vi "py.vi"() -> ()   [LabVIEW 2023]
panel:
  in  "x 2":dbl(slide) scale=0.0..10.0
  in  "Stop":bool
  out "Numeric":i32
  out "return value":T1
  in  "x":dbl(slide) scale=0.0..10.0
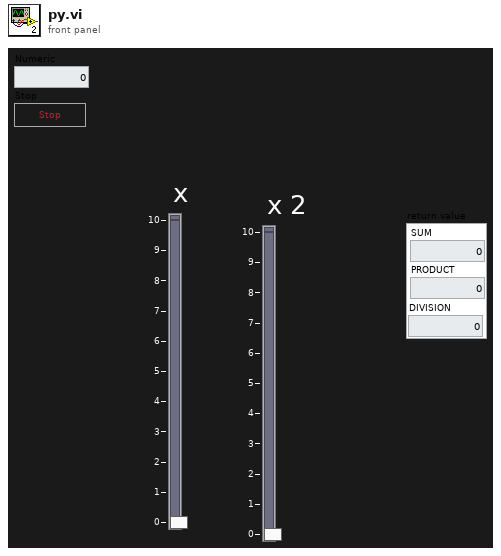
[diagram p1: front panel]
types:
  T1 = cluster{"SUM":dbl, "PRODUCT":dbl, "DIVISION":dbl}
  T2 = cluster{"Numeric":dbl, "Numeric 2":dbl, "Numeric 3":dbl}
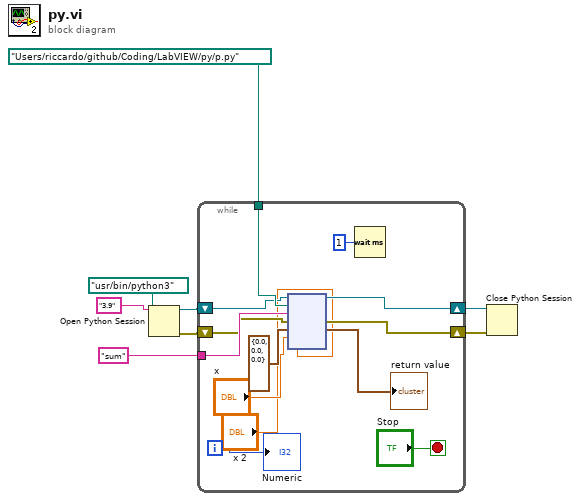
[diagram p0: block diagram]
diagram:
  n1 = Open Python Session(python version="3.9" ("Python version"), python path=path "/usr/bin/python3" ("Python path")) -> (session out=w6:refnum<k35>, error out=w2:errorcluster)  [unwired: 1 in]
  n2 = while {
    tunnel: path "/Users/riccardo/github/Coding/LabVIEW/py/p.py" ("Path") -> [w21]
    tunnel: "sum" ("function name") -> [w19]
    shift-right: [w18] -> w4
    shift-left: w6 -> [w20]
    shift-right: [w17] -> w3
    shift-left: w2 -> [w16]
    i -> [w13]
    stop <- "Stop" stop-if-true
    n3 = node(w20, w21, w19, w16, T2 {"Numeric"=0.0, "Numeric 2"=0.0, "Numeric 3"=0.0} ("Cluster"), "x", "x 2") -> (w18:refnum<k35>, w17:errorcluster, →"return value":T2)  [unwired: 2 in, 2 out]
    n4 = Wait (ms)(milliseconds to wait=u32 1) -> ()  [unwired: 1 out]
    "Numeric" <- w13
  }
  n5 = Close Python Session(session in=w4, error in=w3) -> ()  [unwired: 1 out]
